vi "dds_host_new.vi"() -> ()   [LabVIEW 2018]
uses:
  <vilib>/rvi/Analysis/host/Butterworth/config/Butterworth Filter Order.ctl
  <vilib>/rvi/Analysis/host/Butterworth/config/Butterworth Filter Type.ctl
  <vilib>/FPGAPlugInAG/PCIe-7841R/niLvFpga_Open_PCIe-7841R.vi
  <vilib>/rvi/interface/common/dynamic/niFpgaDynamicAddResources.vi
  <vilib>/FPGAPlugInAG/Dynamic/niLvFpga_Run_Dynamic.vi
  <vilib>/rvi/Analysis/host/Butterworth/config/BwScaledCoefficients.vi
  <vilib>/Utility/error.llb/Error Cluster From Error Code.vi
  <vilib>/rvi/errors/niLvFpgaAdjustHostInterfaceError.vi
  <vilib>/FPGAPlugInAG/Dynamic/niLvFpga_Close_Dynamic.vi
  <vilib>/rvi/interface/nirviOpenFPGA/nirviOpenFPGA.xnode
  FPGA Bitfiles/dds_FPGATarget_ddsfpganew_7EP1GNzA9aI.lvbitx
  <vilib>/rvi/interface/nirviMethod/nirviMethod.xnode
  <vilib>/rvi/Analysis/host/Butterworth/XNode/ButterworthCoefficients.xnode
  <vilib>/rvi/interface/nirviReadWriteControl/nirviReadWriteControl.xnode
  <vilib>/rvi/interface/nirviCloseFPGA/nirviCloseFPGA.xnode
  <vilib>/rvi/Analysis/host/Public/NI_FpgaMspHost.lvlib
  NiFpgaLv.dll
  <vilib>/rvi/interface/Simulation/niFpgaSimulationCallBeginRW.vi
panel:
  in  "reset phi sum":bool
  in  "reset sig sum":bool
  out "host rate":dbl=500.0
  in  "subtract phi mean":bool=TRUE
  in  "stop dds":bool
  in  "phi_pg":fxp<+/-,16,8>
  out "phi_dc_offset":fxp<+,32,0>=0.5
  out "downsample_fifo_write_time":u32=50
  out "fb_fifo_timeout":bool
  in  "desired feedback loop time":u32=50
  out "feedback loop time":u32=50
  out "cross_pol_phi_shifted":dbl(graph)=216.255859375
  out "phi_dg":fxp<+/-,16,8>
  in  "phase_mod_offset":fxp<+,32,0>=0.5
  in  "user_phi_dc_offset":fxp<+,32,0>=0.5
  in  "phi_upper_lim":fxp<+/-,32,0>=0.49999999976716936
  in  "phi_lower_lim":fxp<+/-,32,0>=-0.5
  in  "user_phi_dg":fxp<+/-,16,8>
  in  "phi_set":fxp<+/-,32,16>
  out "scaled_noise":dbl(graph)
  in  "noise_scale":fxp<+,32,0>=0.010000000009313226
  in  "phase_mod_scale":fxp<+,16,0>
  out "analog fsamp":dbl=200000.00000000003 format="%#_6p"
  in  "high pass cutoff":dbl=46000.0
  in  "low pass cutoff":dbl=54000.0
  in  "reset filters?":bool
  out "synth_settings_client":dbl[](array[numeric])=[1.0, 25000.0, 10.0, 0.0234375, 0.5]
  out "error out":errorcluster={"status"=FALSE, "code"=61003, "source"="niLvFpga_Run_Dynamic.vi"}
  in  "stop host":bool
  in  "step_time (ms)":u32=2
  in  "re-initialize_dds":bool
  out "Actual Sample Rate (S/s)":dbl=952380.9523809524 format="%#_6p"
  out "Sampling Rate\nAchieved?":bool=TRUE
  out "requested_freq":dbl(graph)=25000.0
  in  "Desired loop rate (ticks)":u32=84
  in  "vpp 01":dbl
  in  "vpp 23":dbl
  in  "vpp 45":dbl
  in  "set xy drive":bool
  out "scale factor 01":fxp<+/-,16,1>
  out "scale factor 23":fxp<+/-,16,1>=0.04998779296875
  out "scale factor 45":fxp<+/-,16,1>=0.04998779296875
  in  "just x?":bool
  in  "01_sin":bool=TRUE
  in  "23_sin":bool
  in  "45_sin":bool=TRUE
  in  "z_slow-dds?":bool
  in  "slow-dds_param":T1={"Sine wave frequency (Hz)"=25.0, "Phase offset (deg)"=0.0} {"Phase offset (deg)" format="%#_6p"; "Sine wave frequency (Hz)" format="%#_6p"}
  in  "vpp_slow-dds":dbl
  out "scale factor_slow-dds":fxp<+/-,16,1>
  out "slow_freq":dbl=25.0
  in  "subtract_mean?":bool=TRUE
  out "cross_pol_amp":dbl(graph)=529.7707061767578
  in  "counter_offset":u8
  in  "discont_neg":fxp<+/-,64,32>=-1.0
  in  "discont_pos":fxp<+/-,17,3>=1.0
  in  "reset_phi":bool
  in  "desired_AI_loop_time(uSec)":u32=5
  out "actual_analog_in_loop_time":u32=5
  out "cross_pol_phi":dbl(graph)=93.5540771484375
  in  "downsample_num":i16=10
  in  "fast-dds_param":T1={"Sine wave frequency (Hz)"=41.0, "Phase offset (deg)"=180.0} {"Phase offset (deg)" format="%#_6p"; "Sine wave frequency (Hz)" format="%#_6p"}
  in  "phase_mod_param":T1={"Sine wave frequency (Hz)"=10.0, "Phase offset (deg)"=0.0} {"Phase offset (deg)" format="%#_6p"; "Sine wave frequency (Hz)" format="%#_6p"}
  out "phase_mod_out":dbl(graph)=0.5
  in  "phase_mod":bool
  in  "initialize_phase_mod":bool
  in  "phi_bitshift":i16=8
  out "phi_fb_out":dbl(graph)=0.5
  in  "test_phase_mod":bool
  in  "change_pm_freq":bool
  in  "frequency increment":dbl=0.2
  in  "change_phi_dg":bool
  in  "xy_amplitude_mod?":bool
  in  "sine_amp":dbl format="%#_13g"
  in  "frequency":u32=100
  in  "reset_accum":bool
  out "In Range?":bool=TRUE
  out "amplitude_modulation":dbl(graph)=-0.0
  in  "noise":bool
  in  "RMS":u16=4096
  in  "change_phi_offset":bool
  in  "set yz drive":bool
  in  "set xz drive":bool
types:
  T1 = cluster{"Sine wave frequency (Hz)":dbl, "Phase offset (deg)":dbl}
  T2 = enum16{"open", "replace", "create", "open or create", "replace or create", "replace or create with confirmation"}
  T3 = cluster{"frequency (periods/tick)":fxp<+,32,0>, "phase offset (periods)":fxp<+,32,0>, fxp<+/-,16,1>, fxp<+,1,1>}
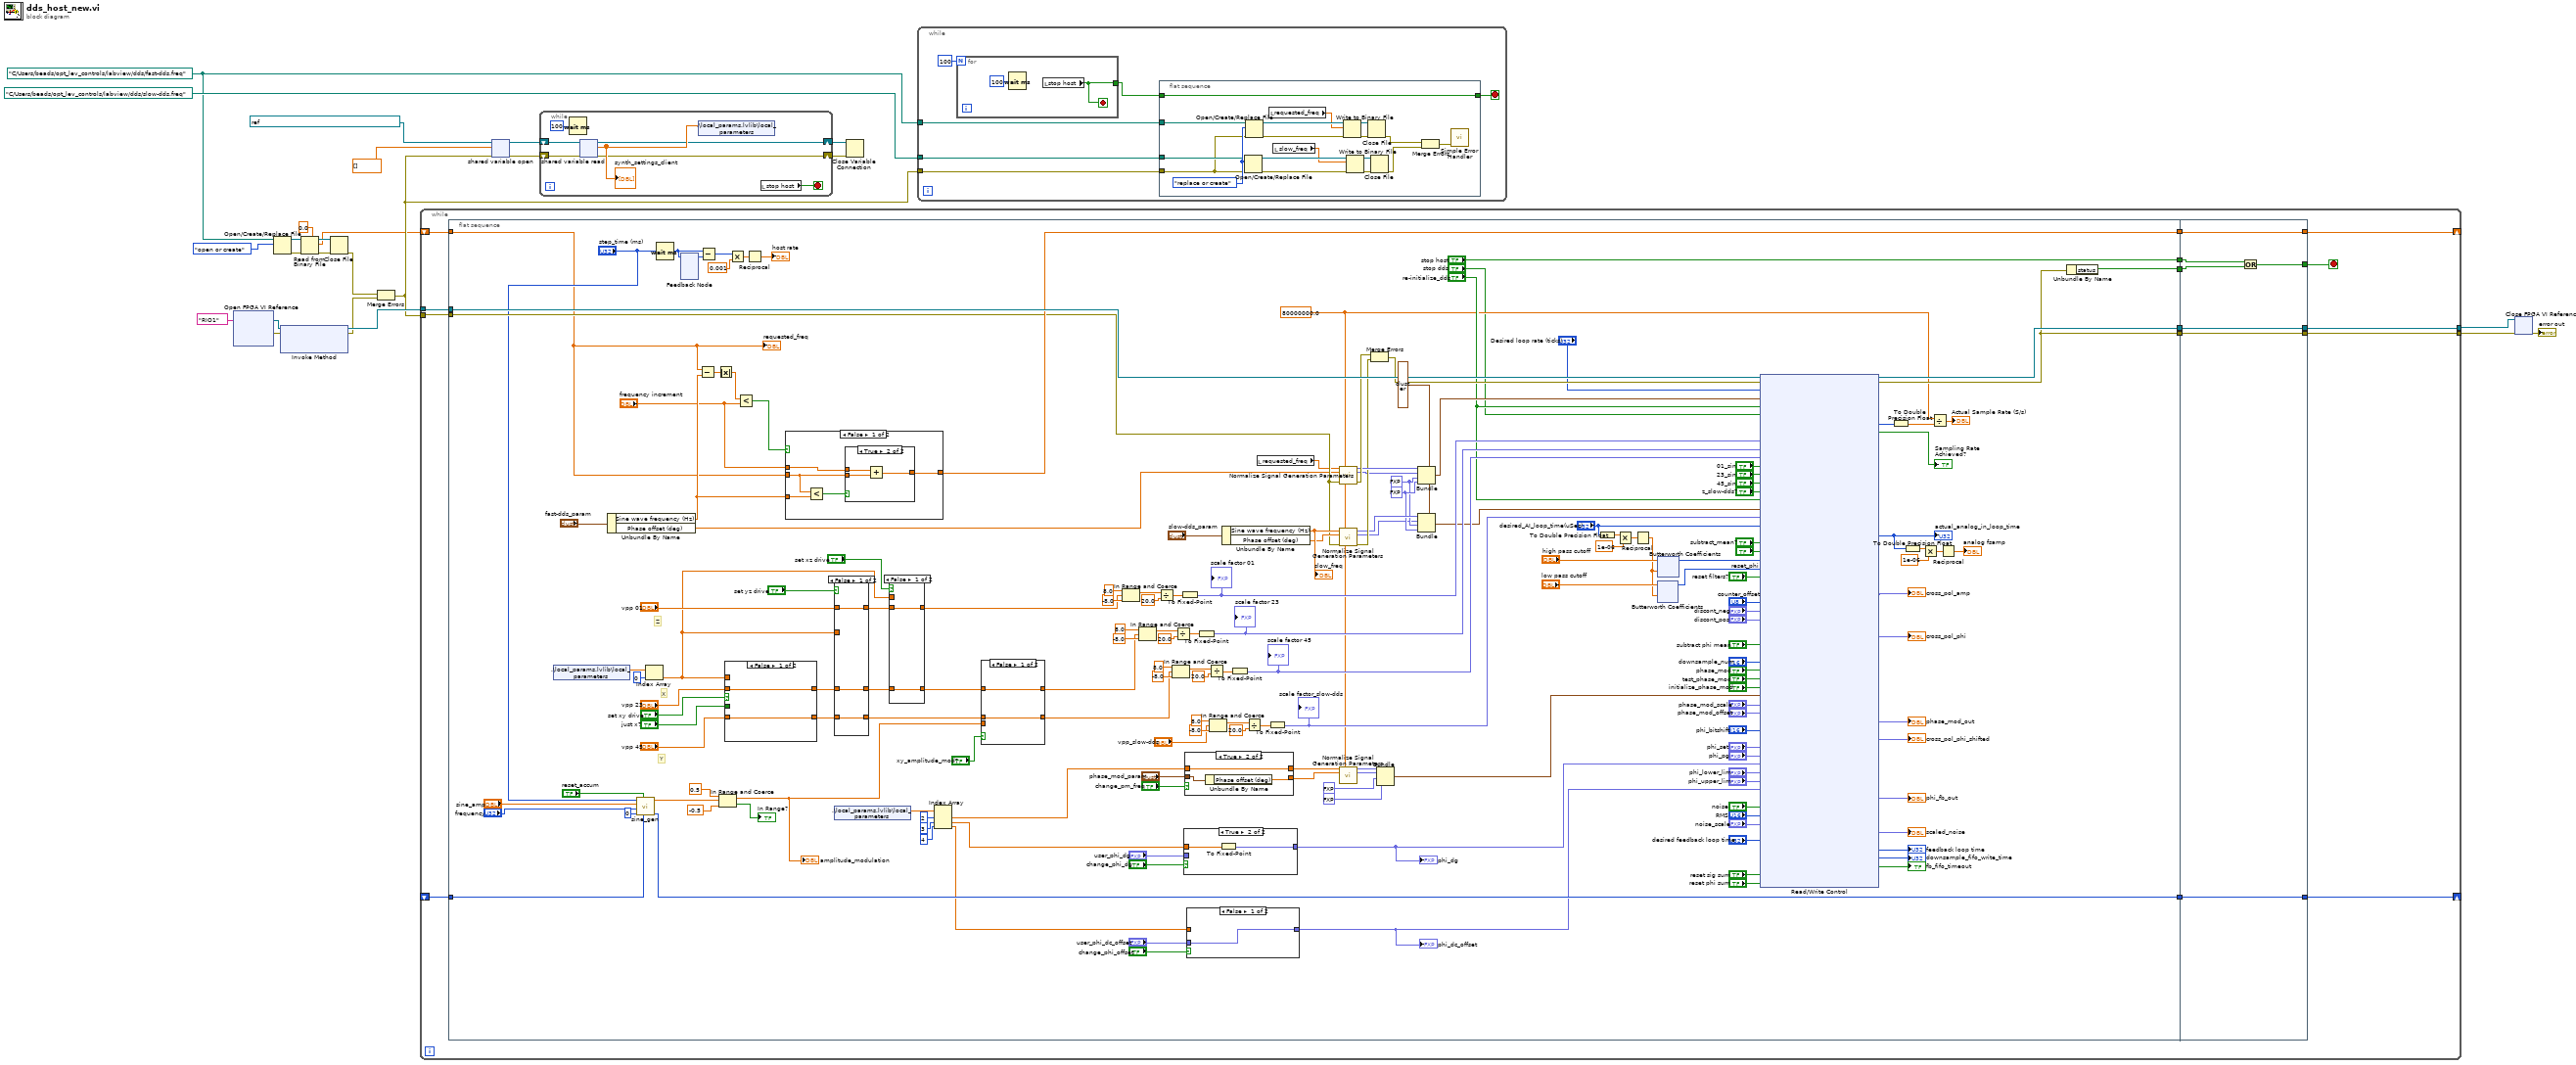
[diagram p0: block diagram]
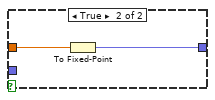
[diagram p4: hidden frame]
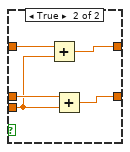
[diagram p5: hidden frame]
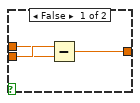
[diagram p7: hidden frame]
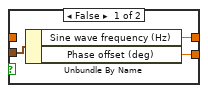
[diagram p9: hidden frame]
diagram:
  w13 = path "C:/Users/beads/opt_lev_controls/labview/dds/fast-dds.freq" ("file path (use dialog)")
  n1 = xnode "Open FPGA VI Reference"("resource name"=tag "RIO1") -> ("FPGA VI Reference Out"=w23:refnum<k20>, "error out"=w24:errorcluster)  [unwired: 1 in]
  n2 = Open/Create/Replace File(file path (use dialog)=w13, operation (0:open)=T2."open or create") -> (refnum out=w11:refnum<file>, error out=w12:errorcluster)  [unwired: 4 in, 1 out]
  n3 = xnode "Invoke Method"("FPGA VI Reference In"=w23, "error in"=w24) -> ("FPGA VI Reference Out"=w22:refnum<k20>, "error out"=w8:errorcluster)  [unwired: 1 in]
  n4 = Read from Binary File(5:0.0, 8:w12, 11:w11) -> (0:w10:errorcluster, 2:w3:dbl, 3:w9:refnum<file>)  [unwired: 3 in, 1 out]
  n5 = Close File(refnum=w9, error in=w10) -> (error out=w7:errorcluster)  [unwired: 1 out]
  n6 = Merge Errors(w7, w8) -> (w4:errorcluster)
  n7 = while {
    tunnel: w22 -> [w40]
    tunnel: w4 -> [w36]
    tunnel: [w38] -> w2
    tunnel: [w39] -> w1
    shift-right: [w37] -> _
    shift-left: w3 -> [w33]
    shift-right: [w35] -> _
    shift-left: _ -> [w34]
    stop <- w26 stop-if-true
    n8 = flat-sequence {
      tunnel: w40 -> [w215]
      tunnel: w36 -> [w169]
      tunnel: w34 -> [w116]
      tunnel: w33 -> [w109]
      tunnel: [w214] -> w32
      tunnel: [w213] -> w31
      tunnel: [w212] -> w30
      tunnel: ["stop host"] -> w29
      tunnel: [w194] -> w28
      tunnel: [w117] -> w27
      tunnel: [w280] -> w35
      tunnel: [w281] -> w37
      tunnel: [w282] -> w38
      tunnel: [w283] -> w39
      tunnel: w32 -> [w283]
      tunnel: w31 -> [w282]
      tunnel: w30 -> [w279]
      tunnel: w29 -> [w278]
      tunnel: w28 -> [w281]
      tunnel: w27 -> [w280]
      tunnel: [w277] -> w26
      frame #0 {
        w164 = fxp<+/-,16,1> 0.0
        w167 = T3 {"frequency (periods/tick)"=0.0, "phase offset (periods)"=0.0, 0.0, 0.0} ("cluster")
        w165 = fxp<+,1,1> 0.0
        w142 = 80000000.0 ("FPGA clock rate (Hz)")
        # "Y"
        # "X"
        # "Z"
        n9 = shared-variable ".\\local_params.lvlib\\local_parameters"() -> (w193:dbl[])  [unwired: 1 in, 1 out]
        n10 = Unbundle By Name("fast-dds_param") -> ("Sine wave frequency (Hz)"=w198:dbl, "Phase offset (deg)"=w148:dbl)
        n11 = call "sine_gen.vi"("prev_val"=w116, "reset_accum"="reset_accum", "phase_shift 2"=u32 0, "frequency"="frequency", "sine_amp"="sine_amp", "step_time(ms)"="step_time (ms)") -> ("next_val"=w117:u32, "sine_out"=w111:dbl)  [unwired: 3 in]
        n12 = Index Array(array=w193, index=0) -> (element=w102:dbl)
        n13 = Wait (ms)(milliseconds to wait="step_time (ms)") -> (millisecond timer value=w48:u32)
        n14 = feedback #1() -> (w47:u32)  [unwired: 1 in]
        n15 = feedback-in #1(w48) -> ()
        n16 = Subtract(x=w109, y=w198) -> (x-y=w132:dbl)
        n17 = Subtract(x=w48, y=w47) -> (x-y=w46:u32)
        n18 = Absolute Value(x=w132) -> (abs(x)=w131:dbl)
        n19 = In Range and Coerce(upper limit=0.5, x=w111, lower limit=-0.5) -> (coerced(x)=w112:dbl, In Range?=→"In Range?":bool)
        "amplitude_modulation" <- w112
        n20 = case shown="False" "set xy drive" {
          tunnel: "vpp 23" -> [w270 _]
          tunnel: [w270 w271] -> w105
          tunnel: "vpp 45" -> [w269 w273]
          tunnel: [w269 w272] -> w104
          tunnel: "just x?" -> [_ w274]
          tunnel: w102 -> [_ w271]
          frame False {
          }
          frame True {
            n21 = case shown="False" w274 {
              tunnel: w273 -> [_ w276]
              tunnel: [w275 w276] -> w272
              tunnel: w271 -> [w275 _]
              frame False {
              }
              frame True {
              }
            }
          }
        }
        n22 = Multiply(x=w46, y=0.001) -> (x*y=w44:dbl)
        n23 = Less?(x=w131, y="frequency increment") -> (x < y?=w129:bool)
        n24 = Reciprocal(x=w44) -> (1/x=→"host rate":dbl)
        n25 = case shown="False" w129 {
          tunnel: [w252 w262] -> w194
          tunnel: w109 -> [w251 _]
          tunnel: w198 -> [w255 w262]
          tunnel: "frequency increment" -> [w253 _]
          frame False {
            n26 = Less?(x=w251, y=w255) -> (x < y?=w254:bool)
            n27 = case shown="True" w254 {
              tunnel: w251 -> [w257 w261]
              tunnel: w253 -> [w256 w260]
              tunnel: [w258 w259] -> w252
              frame False {
                n28 = Subtract(x=w257, y=w256) -> (x-y=w258:dbl)
              }
              frame True {
                n29 = Add(x=w260, y=w261) -> (x+y=w259:dbl)
              }
            }
          }
          frame True {
          }
        }
        n30 = case shown="False" "set yz drive" {
          tunnel: [w235 w237] -> w101
          tunnel: "vpp 01" -> [w235 _]
          tunnel: w102 -> [_ w237]
          tunnel: [w234 w236] -> w98
          tunnel: w105 -> [w234 w236]
          tunnel: [w233 w237] -> w97
          tunnel: w104 -> [w233 _]
          frame False {
          }
          frame True {
          }
        }
        n31 = shared-variable ".\\local_params.lvlib\\local_parameters"() -> (w135:dbl[])  [unwired: 1 in, 1 out]
        n32 = case shown="False" "set xz drive" {
          tunnel: w102 -> [_ w232]
          tunnel: w101 -> [w231 _]
          tunnel: [w231 w232] -> w100
          tunnel: [w230 w232] -> w99
          tunnel: w98 -> [w230 _]
          frame False {
          }
          frame True {
          }
        }
        n33 = Index Array(array=w135, index #1=2 ("index"), index #2=3 ("index"), index #3=4 ("index")) -> (element #1=w133:dbl, element #2=w127:dbl, element #3=w53:dbl)
        n34 = case shown="False" "xy_amplitude_mod?" {
          tunnel: w99 -> [w242 w247]
          tunnel: [w242 w245] -> w125
          tunnel: w97 -> [w241 w246]
          tunnel: [w241 w244] -> w124
          tunnel: w112 -> [_ w243]
          frame False {
          }
          frame True {
            n35 = Add(x=w247, y=w243) -> (x+y=w245:dbl)
            n36 = Add(x=w246, y=w243) -> (x+y=w244:dbl)
          }
        }
        n37 = In Range and Coerce(upper limit=8.0, x=w100, lower limit=-8.0) -> (coerced(x)=w201:dbl)  [unwired: 1 out]
        n38 = In Range and Coerce(upper limit=8.0, x=w125, lower limit=-8.0) -> (coerced(x)=w182:dbl)  [unwired: 1 out]
        n39 = Divide(x=w201, y=20.0) -> (x/y=w207:dbl)
        n40 = In Range and Coerce(upper limit=8.0, x=w124, lower limit=-8.0) -> (coerced(x)=w176:dbl)  [unwired: 1 out]
        n41 = Divide(x=w182, y=20.0) -> (x/y=w183:dbl)
        n42 = To Fixed-Point(number=w207) -> (fixed-point=w196:fxp<+/-,16,1>)  [unwired: 1 in]
        "scale factor 01" <- w196
        n43 = case shown="True" "change_phi_dg" {
          tunnel: w127 -> [_ w250]
          tunnel: [w248 w249] -> w63
          tunnel: "user_phi_dg" -> [w248 _]
          frame False {
          }
          frame True {
            n44 = To Fixed-Point(number=w250) -> (fixed-point=w249:fxp<+/-,16,8>)  [unwired: 1 in]
          }
        }
        "phi_dg" <- w63
        n45 = case shown="True" "change_pm_freq" {
          tunnel: "phase_mod_param" -> [w265 w268]
          tunnel: [w264 w267] -> w144
          tunnel: [w263 w266] -> w143
          tunnel: w133 -> [_ w267]
          frame False {
            n46 = Unbundle By Name(w265) -> ("Sine wave frequency (Hz)"=w264:dbl, "Phase offset (deg)"=w263:dbl)
          }
          frame True {
            n47 = Unbundle By Name(w268) -> ("Phase offset (deg)"=w266:dbl)
          }
        }
        n48 = case shown="False" "change_phi_offset" {
          tunnel: "user_phi_dc_offset" -> [w238 _]
          tunnel: w53 -> [_ w240]
          tunnel: [w238 w239] -> w52
          frame False {
          }
          frame True {
            n49 = To Fixed-Point(number=w240) -> (fixed-point=w239:fxp<+,32,0>)  [unwired: 1 in]
          }
        }
        "phi_dc_offset" <- w52
        n50 = To Fixed-Point(number=w183) -> (fixed-point=w179:fxp<+/-,16,1>)  [unwired: 1 in]
        "scale factor 23" <- w179
        n51 = Divide(x=w176, y=20.0) -> (x/y=w177:dbl)
        n52 = In Range and Coerce(upper limit=8.0, x="vpp_slow-dds", lower limit=-8.0) -> (coerced(x)=w160:dbl)  [unwired: 1 out]
        n53 = Unbundle By Name("slow-dds_param") -> ("Sine wave frequency (Hz)"=w171:dbl, "Phase offset (deg)"=w170:dbl)
        "slow_freq" <- w171
        n54 = To Fixed-Point(number=w177) -> (fixed-point=w173:fxp<+/-,16,1>)  [unwired: 1 in]
        "scale factor 45" <- w173
        n55 = Divide(x=w160, y=20.0) -> (x/y=w161:dbl)
        n56 = local read "requested_freq"() -> (w96:dbl)
        n57 = To Fixed-Point(number=w161) -> (fixed-point=w156:fxp<+/-,16,1>)  [unwired: 1 in]
        "scale factor_slow-dds" <- w156
        n58 = call <vilib>:"Normalize Signal Generation Parameters.vi"("frequency (Hz)"=w96, "FPGA clock rate (Hz)"=w142, "phase offset (deg)"=w148, "error in (no error)"=w169) -> ("frequency (periods/tick)"=w209:fxp<+,32,0>, "phase offset (periods)"=w146:fxp<+,32,0>, "error out"=w211:errorcluster)  [unwired: 6 in, 3 out]
        n59 = call <vilib>:"Normalize Signal Generation Parameters.vi"("frequency (Hz)"=w171, "FPGA clock rate (Hz)"=w142, "phase offset (deg)"=w170, "error in (no error)"=w169) -> ("frequency (periods/tick)"=w166:fxp<+,32,0>, "phase offset (periods)"=w147:fxp<+,32,0>, "error out"=w168:errorcluster)  [unwired: 6 in, 3 out]
        n60 = call <vilib>:"Normalize Signal Generation Parameters.vi"("frequency (Hz)"=w144, "FPGA clock rate (Hz)"=w142, "phase offset (deg)"=w143) -> ("frequency (periods/tick)"=w141:fxp<+,32,0>, "phase offset (periods)"=w140:fxp<+,32,0>)  [unwired: 7 in, 4 out]
        n61 = Merge Errors(w211, w168) -> (w210:errorcluster)
        n62 = Bundle("frequency (periods/tick)"=w141, "phase offset (periods)"=w140, fxp<+/-,16,1> 0.0, fxp<+,1,1> 0.0) -> (w65:T3)  [unwired: 1 in]
        n63 = Bundle(cluster=w167, "frequency (periods/tick)"=w209, "phase offset (periods)"=w146, w164, w165) -> (w206:T3)
        n64 = Bundle(cluster=w167, "frequency (periods/tick)"=w166, "phase offset (periods)"=w147, w164, w165) -> (w163:T3)
        n65 = To Double Precision Float(number="desired_AI_loop_time(uSec)") -> (double precision float=w88:dbl)
        n66 = Multiply(x=w88, y=1e-06) -> (x*y=w87:dbl)
        n67 = Reciprocal(x=w87) -> (1/x=w89:dbl)
        n68 = xnode "Butterworth Coefficients"("cutoff frequency (Hz)"="low pass cutoff", "sample rate (S/s)"=w89) -> ("scaled coefficients"=w94:i32[])  [unwired: 1 in, 1 out]
        n69 = xnode "Butterworth Coefficients"("cutoff frequency (Hz)"="high pass cutoff", "sample rate (S/s)"=w89) -> ("scaled coefficients"=w92:i32[])  [unwired: 1 in, 1 out]
        n70 = xnode "Read/Write Control"("FPGA VI Reference In"=w215, "error in"=w210, "Desired loop rate (ticks)"="Desired loop rate (ticks)", "sinewave-props_fast-dds"=w206, "Initialize fast-dds"="re-initialize_dds", "stop"="stop dds", "fast-dds_scale01"=w196, "fast-dds_scale23"=w179, "fast-dds_scale45"=w173, "01_sin"="01_sin", "23_sin"="23_sin", "45_sin"="45_sin", "z_slow-dds?"="z_slow-dds?", "Initialize slow-dds"="re-initialize_dds", "sinewave-props_slow-dds"=w163, "slow-dds_scale"=w156, "desired_analog_in_loop_time_(uSec)"="desired_AI_loop_time(uSec)", "subtract_mean"="subtract_mean?", "reset_phi"="reset_phi", "high pass butter coeff"=w92, "low pass butter coeff"=w94, "reset filters?"="reset filters?", "counter_offset"="counter_offset", "discont_neg"="discont_neg", "discont_pos"="discont_pos", "subtract phi mean"="subtract phi mean", "downsample_num"="downsample_num", "phase_mod"="phase_mod", "test_phase_mod"="test_phase_mod", "initialize_phase_mod"="initialize_phase_mod", "phase_mod_props"=w65, "phase_mod_scale"="phase_mod_scale", "phase_mod_offset"="phase_mod_offset", "phi_bitshift"="phi_bitshift", "phi_set"="phi_set", "phi_pg"="phi_pg", "phi_dg"=w63, "phi_lower_lim"="phi_lower_lim", "phi_upper_lim"="phi_upper_lim", "phi_dc_offset"=w52, "noise"="noise", "RMS"="RMS", "noise_scale"="noise_scale", "desired feedback loop time"="desired feedback loop time", "reset sig sum"="reset sig sum", "reset phi sum"="reset phi sum") -> ("FPGA VI Reference Out"=w214:refnum<k20>, "error out"=w213:errorcluster, "Actual loop rate"=w203:u32, "Sampling rate achieved?"=→"Sampling Rate\nAchieved?":bool, "actual_analog_in_loop_time"=w81:u32, "cross_pol_amp"=→"cross_pol_amp":fxp<+,32,16>, "phi_full_out"=→"cross_pol_phi":fxp<+/-,32,18>, "phase_mod_out"=→"phase_mod_out":fxp<+,32,0>, "cross_pol_phi_shifted"=→"cross_pol_phi_shifted":fxp<+/-,32,16>, "phi_fb_out"=→"phi_fb_out":fxp<+,32,0>, "scaled noise"=→"scaled_noise":fxp<+/-,32,0>, "feedback loop time"=→"feedback loop time":u32, "downsample_fifo_write_time"=→"downsample_fifo_write_time":u32, "fb_fifo_timeout"=→"fb_fifo_timeout":bool)  [unwired: 3 out]
        "actual_analog_in_loop_time" <- w81
        n71 = To Double Precision Float(number=w203) -> (double precision float=w205:dbl)
        n72 = To Double Precision Float(number=w81) -> (double precision float=w85:dbl)
        n73 = Multiply(x=w85, y=1e-06) -> (x*y=w84:dbl)
        n74 = Divide(x=w142, y=w205) -> (x/y=→"Actual Sample Rate (S/s)":dbl)
        n75 = Reciprocal(x=w84) -> (1/x=→"analog fsamp":dbl)
        n76 = Unbundle By Name(w213) -> ("status"=w212:bool)
        "requested_freq" <- w109
      }
      frame #1 {
        n77 = Or(x=w278, y=w279) -> (x .or. y?=w277:bool)
      }
    }
  }
  n78 = shared-variable-open(refnum<k21> "ni.var.psp://localhost/daq_lib/synth_settings" ("shared variable refnum in"), w4, dbl[] [] ("synth_settings_client")) -> (w18:refnum<k21>, w17:errorcluster)  [unwired: 1 in]
  n79 = while {
    shift-right: [w285] -> w16
    shift-left: w18 -> [w288]
    shift-right: [w284] -> w15
    shift-left: w17 -> [w287]
    stop <- w289 stop-if-true
    n80 = Wait (ms)(milliseconds to wait=u32 100) -> ()  [unwired: 1 out]
    n81 = shared-variable-read(w288, w287) -> (w285:refnum<k21>, w284:errorcluster, w286:dbl[])  [unwired: 1 out]
    "synth_settings_client" <- w286
    n82 = shared-variable ".\\local_params.lvlib\\local_parameters"(w286) -> ()  [unwired: 1 in, 1 out]
    n83 = local read "stop host"() -> (w289:bool)
  }
  n84 = Close Variable Connection(8:w15, 11:w16) -> ()  [unwired: 1 out]
  n85 = while {
    tunnel: w13 -> [w296]
    tunnel: path "C:/Users/beads/opt_lev_controls/labview/dds/slow-dds.freq" ("file path (use dialog)") -> [w295]
    tunnel: w4 -> [w293]
    stop <- w291 stop-if-true
    n86 = for {
      N: 100 -> [_]
      tunnel: [w316] -> w292
      stop <- w316 stop-if-true
      n87 = Wait (ms)(milliseconds to wait=u32 100) -> ()  [unwired: 1 out]
      n88 = local read "stop host"() -> (w316:bool)
    }
    n89 = flat-sequence {
      tunnel: w296 -> [w300]
      tunnel: w295 -> [w299]
      tunnel: w293 -> [w298]
      tunnel: w292 -> [w297]
      tunnel: [w297] -> w291
      frame #0 {
        w314 = T2."replace or create" ("operation (0:open)")
        n90 = Open/Create/Replace File(file path (use dialog)=w299, error in=w298, operation (0:open)=w314) -> (refnum out=w309:refnum<file>, error out=w310:errorcluster)  [unwired: 3 in, 1 out]
        n91 = Open/Create/Replace File(file path (use dialog)=w300, error in=w298, operation (0:open)=w314) -> (refnum out=w313:refnum<file>, error out=w312:errorcluster)  [unwired: 3 in, 1 out]
        n92 = local read "requested_freq"() -> (w311:dbl)
        n93 = local read "slow_freq"() -> (w308:dbl)
        n94 = Write to Binary File(file (use dialog)=w313, data=w311, error in=w312) -> (refnum out=w306:refnum<file>, error out=w307:errorcluster)  [unwired: 3 in, 1 out]
        n95 = Write to Binary File(file (use dialog)=w309, data=w308, error in=w310) -> (refnum out=w305:refnum<file>, error out=w304:errorcluster)  [unwired: 3 in, 1 out]
        n96 = Close File(refnum=w306, error in=w307) -> (error out=w303:errorcluster)  [unwired: 1 out]
        n97 = Close File(refnum=w305, error in=w304) -> (error out=w302:errorcluster)  [unwired: 1 out]
        n98 = Merge Errors(w303, w302) -> (w301:errorcluster)
        n99 = call <vilib>:"Simple Error Handler.vi"("error in (no error)"=w301) -> ()  [unwired: 4 in, 5 out]
      }
    }
  }
  n100 = xnode "Close FPGA VI Reference"("FPGA VI Reference In"=w1, "error in"=w2) -> ("error out"=→"error out":errorcluster)
